vi "IIR Calculator.vi"() -> ()   [LabVIEW 2017]
uses:
  <vilib>/Analysis/3filter.llb/Filter Passband Type.ctl
  <vilib>/Analysis/3filter.llb/Chebyshev Filter (DBL).vi
  <vilib>/Analysis/3filter.llb/Butterworth Filter (DBL).vi
  <vilib>/Analysis/3filter.llb/Elliptic Filter (DBL).vi
  <vilib>/measure/NI_MAPro.lvlib
  <vilib>/Analysis/NI_AALBase.lvlib
panel:
  out "Saving Data 3":bool caption="Saving Data"
  out "Saving Data 2":bool caption="Saving Data"
  out "Saving Data":bool
  in  "?":bool
  out "Eliptical Filter":dbl[](graph)
  out "Eliptical Filter Output":dbl[](array[numeric])
  in  "Eliptical filter type":T1
  in  "Eliptical Order":i32=2
  in  "stopband attenuation (dB)":dbl=60.0 format="%0.2f"
  in  "passband ripple (dB)":dbl=1.0 format="%0.2f"
  in  "Eliptical Filter: fl":dbl=0.125 format="%0.4f"
  in  "Eliptical Filter: fh":dbl=0.45000000000000007 format="%0.2f"
  out "Chebyshev Filter":dbl[](graph)
  out "Chebyshev Filter Output":dbl[](array[numeric])
  in  "Chebyshev filter type":T1
  in  "Chebyshev order":i32=2
  in  "ripple(dB)":dbl=0.1 format="%0.2f"
  in  "Chebyshev: fl":dbl=0.125 format="%0.4f"
  in  "Chebyshev Filter: fh":dbl=0.45000000000000007 format="%0.2f"
  out "Input":waveform(dbl)(graph)
  out "Butterworth Filter":dbl[](graph)
  out "?":dbl[](array[numeric])
  in  "Butterworth filter type":T1
  in  "Butterworth order":i32=2
  in  "Butterworth: fl":dbl=0.12500000000000006 format="%0.4f"
  in  "Butterworth: fh":dbl=0.45000000000000007 format="%0.2f"
  in  "?":string="sin(w*t)*sin(2*pi(1)*t)"
  in  "amplitude":dbl=1.0 format="%0.2p"
  in  "frequency":dbl=10.0 format="%0.2p"
  # "Butterworth Filter Output"
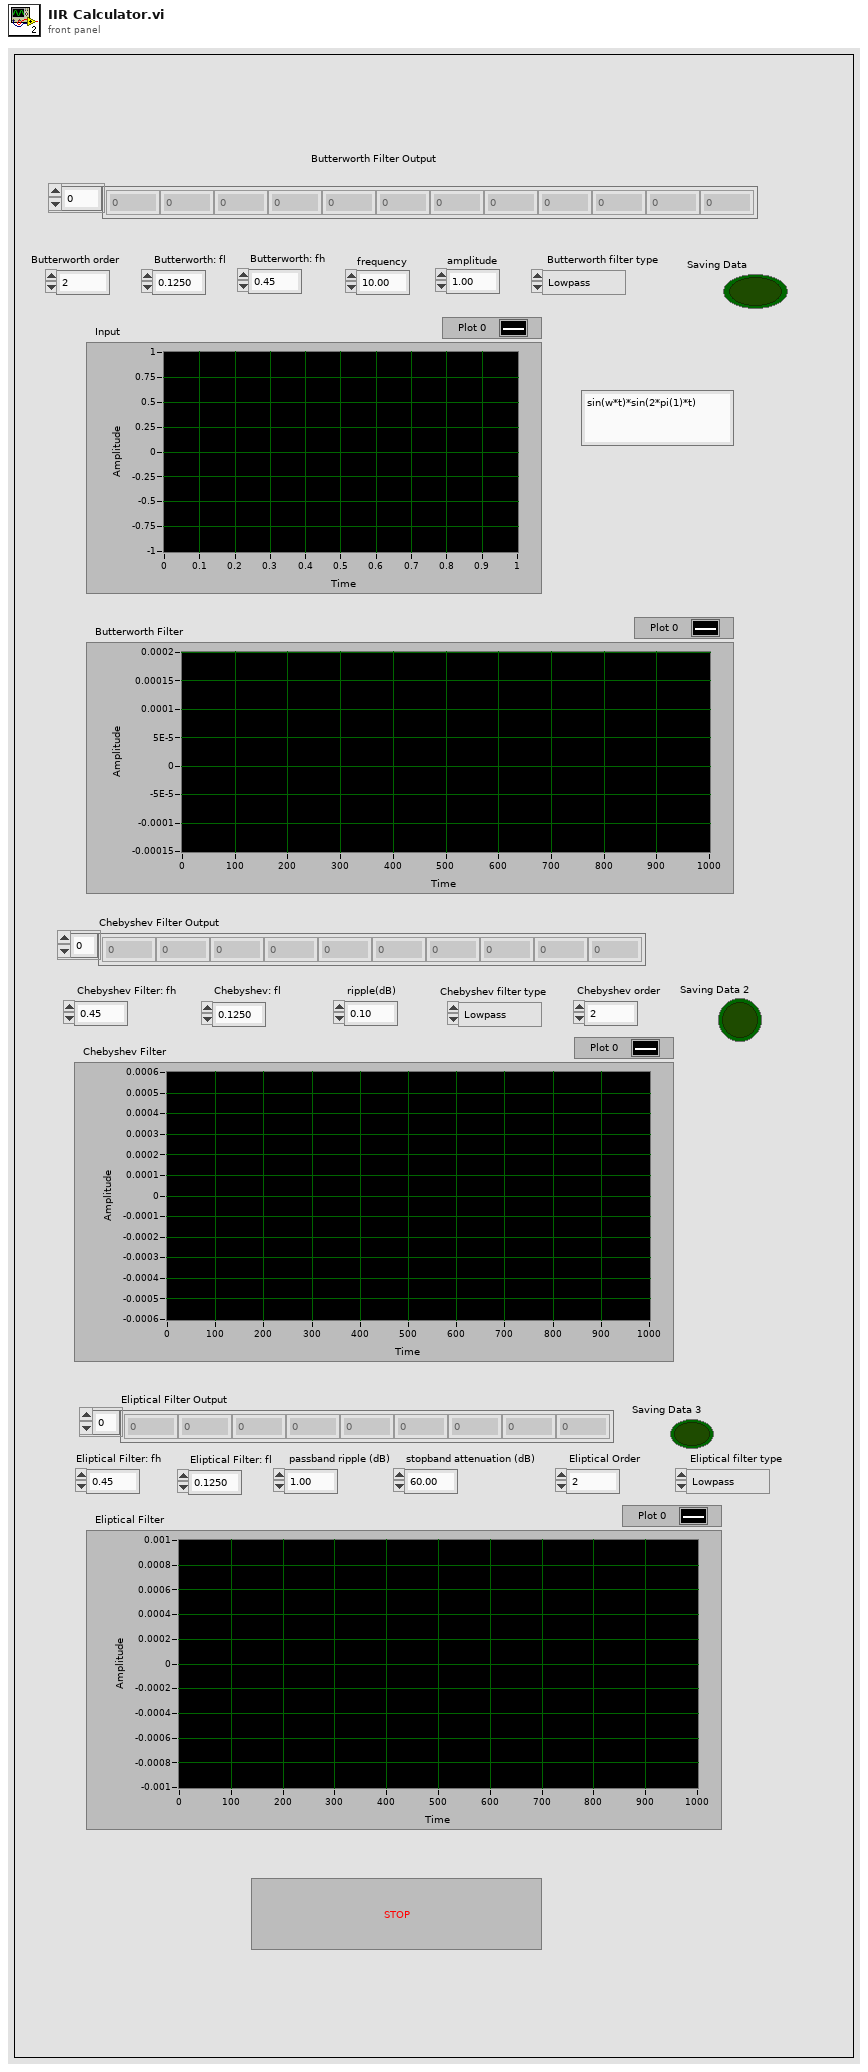
[diagram p1: front panel]
types:
  T1 = typedef "NI_AALBase.lvlib/Filter Passband Type.ctl" = enum32{"Lowpass", "Highpass", "Bandpass", "Bandstop"}
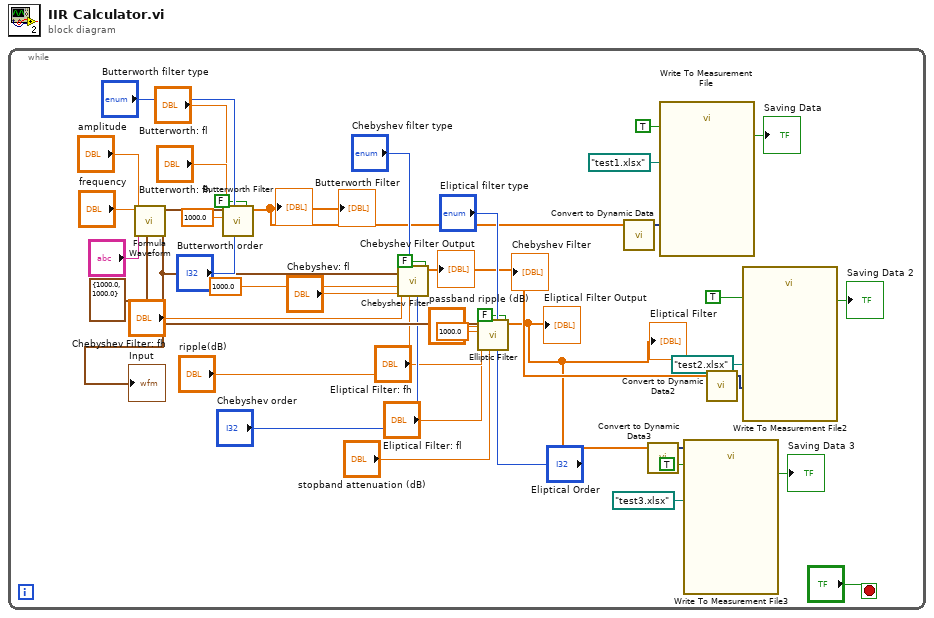
[diagram p0: block diagram]
diagram:
  n1 = while {
    stop <- "?" stop-if-true
    n2 = call <vilib>:"Formula Waveform.vi"("sampling info"=cluster{"Fs":dbl, "#s":dbl} {"Fs"=1000.0, "#s"=1000.0}, "formula"="?", "amplitude"="amplitude", "frequency"="frequency") -> ("signal out"=w33:waveform(dbl))  [unwired: 6 in, 1 out]
    "Input" <- w33
    n3 = call-poly <vilib>:"Butterworth Filter.vi"("init/cont (init:F)"=FALSE, "order"="Butterworth order", "filter type"="Butterworth filter type", "low cutoff freq: fl"="Butterworth: fl", "high cutoff freq: fh"="Butterworth: fh", "sampling freq: fs"=1000.0, "X"=w33) -> ("Filtered X"=w14:dbl[])  [unwired: 1 in, 1 out]
    "?" <- w14
    "Butterworth Filter" <- w14
    n4 = call-poly <vilib>:"Chebyshev Filter.vi"("init/cont (init:F)"=FALSE, "order"="Chebyshev order", "ripple(dB)"="ripple(dB)", "filter type"="Chebyshev filter type", "low cutoff freq: fl"="Chebyshev: fl", "high cutoff freq: fh"="Chebyshev Filter: fh", "sampling freq: fs"=1000.0, "X"=w33) -> ("Filtered X"=w8:dbl[])  [unwired: 2 in, 1 out]
    "Chebyshev Filter Output" <- w8
    "Chebyshev Filter" <- w8
    n5 = call-poly <vilib>:"Elliptic Filter.vi"("init/cont (init:F)"=FALSE, "order"="Eliptical Order", "filter type"="Eliptical filter type", "stopband attenuation (dB)"="stopband attenuation (dB)", "passband ripple (dB)"="passband ripple (dB)", "low cutoff freq: fl"="Eliptical Filter: fl", "high cutoff freq: fh"="Eliptical Filter: fh", "sampling freq: fs"=1000.0, "X"=w33) -> ("Filtered X"=w5:dbl[])  [unwired: 1 in, 1 out]
    "Eliptical Filter Output" <- w5
    "Eliptical Filter" <- w5
    n6 = call "Convert to Dynamic Data"("Array"=w14) -> ("Dynamic Data Type"=w13:dynamicdata)  [unwired: 3 in]
    n7 = call "Convert to Dynamic Data3"("Array"=w5) -> ("Dynamic Data Type"=w4:dynamicdata)  [unwired: 3 in]
    n8 = call "Write To Measurement File"("Signals"=w13, "Enable"=TRUE, "Filename"=path "test1.xlsx") -> ("Saving Data"=→"Saving Data":bool)  [unwired: 14 in, 2 out]
    n9 = call "Write To Measurement File3"("Signals"=w4, "Enable"=TRUE, "Filename"=path "test3.xlsx") -> ("Saving Data"=→"Saving Data 3":bool)  [unwired: 14 in, 2 out]
    n10 = call "Convert to Dynamic Data2"("Array"=w8) -> ("Dynamic Data Type"=w7:dynamicdata)  [unwired: 3 in]
    n11 = call "Write To Measurement File2"("Signals"=w7, "Enable"=TRUE, "Filename"=path "test2.xlsx") -> ("Saving Data"=→"Saving Data 2":bool)  [unwired: 14 in, 2 out]
  }
